vi "To String (Numeric).vi"(7 "enable LabVIEW extensions? (T)":bool=TRUE, 8 "error in (no error)":errorcluster, 11 "JSON Value in":variant) -> (0 "error out":errorcluster, 3 "String":string)   [LabVIEW 2017, in "Advanced Variant Tools.lvlib"]
doc: "Flattens the given JSON data to a string."
uses:
  Advanced Variant Tools.lvlib
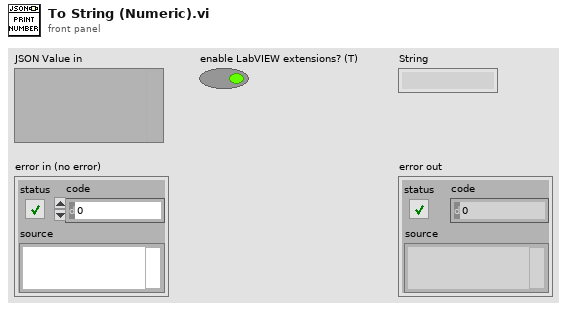
[diagram p1: front panel]
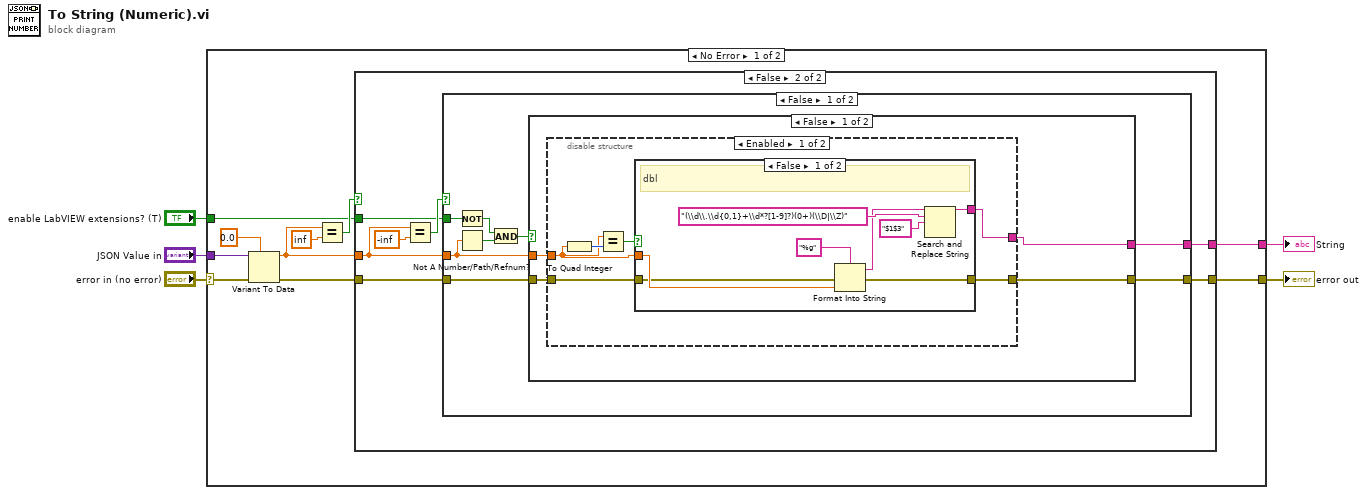
[diagram p0: block diagram]
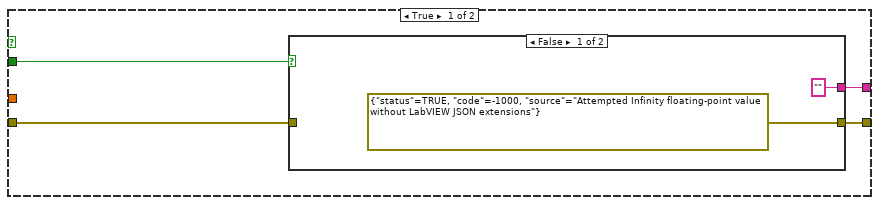
[diagram p2: hidden frame]
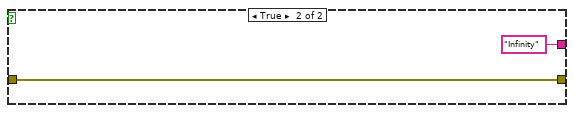
[diagram p3: hidden frame]
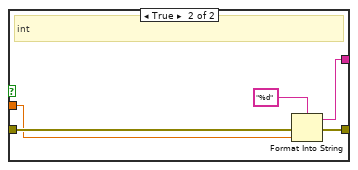
[diagram p4: hidden frame]
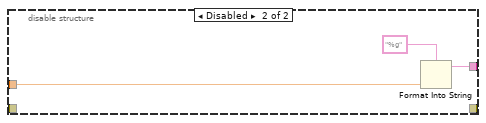
[diagram p5: hidden frame]
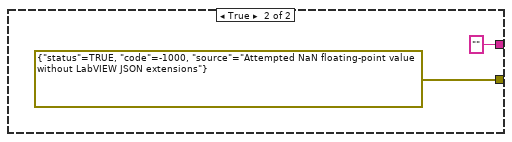
[diagram p6: hidden frame]
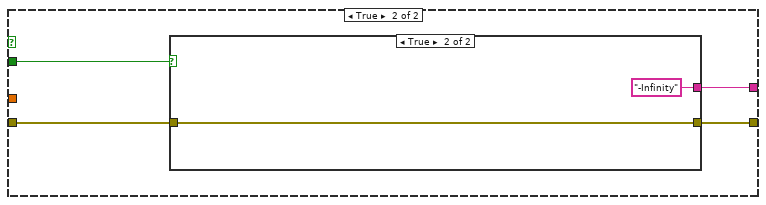
[diagram p7: hidden frame]
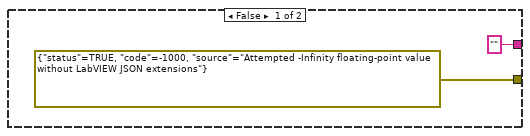
[diagram p8: hidden frame]
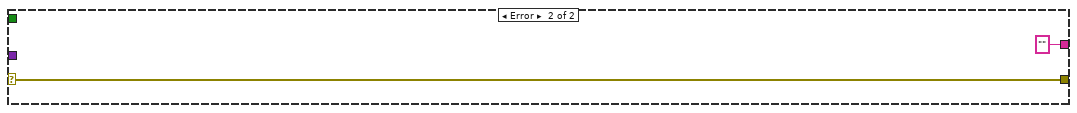
[diagram p9: hidden frame]
diagram:
  n1 = case shown="No Error" "error in (no error)" {
    selector: "error in (no error)" -> [w15 w76]
    tunnel: "JSON Value in" -> [w6 _]
    tunnel: [w14 ""] -> w3
    tunnel: [w13 w76] -> w2
    tunnel: "enable LabVIEW extensions? (T)" -> [w10 _]
    frame No Error {
      n2 = Variant To Data(error in=w15, type=0.0 ("y"), Variant=w6) -> (data=w8:dbl, error out=w9:errorcluster)
      n3 = Equal?(x=w8, y=inf) -> (x = y?=w11:bool)
      n4 = case shown="False" w11 {
        tunnel: w9 -> [w17 w30]
        tunnel: [w19 w29] -> w14
        tunnel: [w16 w28] -> w13
        tunnel: w8 -> [_ w26]
        tunnel: w10 -> [w18 w24]
        frame True {
          n5 = case shown="False" w18 {
            tunnel: ["" "Infinity"] -> w19
            tunnel: w17 -> [_ w22]
            tunnel: [errorcluster {"status"=TRUE, "code"=-1000, "source"="Attempted Infinity floating-point value without LabVIEW JSON extensions"} ("error IO") w22] -> w16
            frame False {
            }
            frame True {
            }
          }
        }
        frame False {
          n6 = Equal?(x=w26, y=-inf) -> (x = y?=w25:bool)
          n7 = case shown="False" w25 {
            tunnel: w30 -> [w38 w68]
            tunnel: [w37 w69] -> w29
            tunnel: [w36 w70] -> w28
            tunnel: w26 -> [w32 _]
            tunnel: w24 -> [w34 w67]
            frame False {
              n8 = Not(x=w34) -> (.not. x?=w33:bool)
              n9 = Not A Number/Path/Refnum?(number/path/refnum=w32) -> (NaN/Path/Refnum?=w31:bool)
              n10 = And(x=w33, y=w31) -> (x .and. y?=w35:bool)
              n11 = case shown="False" w35 {
                tunnel: w38 -> [w42 _]
                tunnel: [w41 ""] -> w37
                tunnel: [w40 errorcluster {"status"=TRUE, "code"=-1000, "source"="Attempted NaN floating-point value without LabVIEW JSON extensions"} ("error IO")] -> w36
                tunnel: w32 -> [w39 _]
                frame False {
                  n12 = disable-structure shown="Enabled" {
                    disable-tunnel: w42 -> [w47 _]
                    disable-tunnel: [w46 w63] -> w41
                    disable-tunnel: [w45 _] -> w40
                    disable-tunnel: w39 -> [w43 w64]
                    frame Enabled {
                      n13 = To Quad Integer(1:w43) -> (0:w44:i64)
                      n14 = Equal?(x=w43, y=w44) -> (x = y?=w48:bool)
                      n15 = case shown="False" w48 {
                        tunnel: w47 -> [w54 w59]
                        tunnel: w43 -> [w56 w57]
                        tunnel: [w49 w60] -> w46
                        tunnel: [w53 w58] -> w45
                        frame False {
                          # "dbl"
                          n16 = Format Into String(format string="%g", error in=w54, w56) -> (resulting string=w50:string, error out=w53:errorcluster)  [unwired: 1 in]
                          n17 = Search and Replace String(input string=w50, search string="(\\d\\.\\d{0,1}+\\d*?[1-9]?)(0+)(\\D|\\Z)", replace string="$1$3" ("replace string (\"\")")) -> (result string=w49:string)  [unwired: 5 in, 3 out]
                        }
                        frame True {
                          # "int"
                          n18 = Format Into String(format string="%d", error in=w59, w57) -> (resulting string=w60:string, error out=w58:errorcluster)  [unwired: 1 in]
                        }
                      }
                    }
                    frame Disabled {
                      n19 = Format Into String(format string="%g", w64) -> (resulting string=w63:string)  [unwired: 2 in, 1 out]
                    }
                  }
                }
                frame True {
                }
              }
            }
            frame True {
              n20 = case shown="True" w67 {
                tunnel: ["" "-Infinity"] -> w69
                tunnel: w68 -> [_ w73]
                tunnel: [errorcluster {"status"=TRUE, "code"=-1000, "source"="Attempted -Infinity floating-point value without LabVIEW JSON extensions"} ("error IO") w73] -> w70
                frame False {
                }
                frame True {
                }
              }
            }
          }
        }
      }
    }
    frame Error {
    }
  }
  "String" <- w3
  "error out" <- w2
